vi "Actor Core.vi"(8 "error in":errorcluster, 11 "Nested in":refnum<class "Messages Actor.lvclass">) -> (0 "error out":errorcluster, 3 "Actor out":refnum<class "Actor.lvclass">)   [LabVIEW 2020, in "Messages Actor.lvlib" / "Messages Actor.lvclass"]
doc: "(<B>Filename</B>: Actor Framework.lvlib:Actor.lvclass:Actor Core.vi)\n\nReceives messages to the actor, reacts to them, and initiates any error handling that may shut the actor down.\n\nDescendant classes may override this VI to append parallel tasks for the actor to complete while it handles messages. Overrides use the Call Parent Method node."
uses:
  Messages Actor.lvclass
  C:/Program Files (x86)/National Instruments/LabVIEW 2020/vi.lib/ActorFramework/Actor/Actor.lvclass
  <vilib>/ActorFramework/Actor/Actor.lvclass
  Controls/Language Enum.ctl
  Messages Actor.lvclass/Messages Actor.ctl
  <vilib>/ActorFramework/Actor/Actor.lvclass/Actor.ctl
  <vilib>/ActorFramework/Message Enqueuer/Message Enqueuer.lvclass/Message Enqueuer.ctl
  Write VI Refnum.vi
  <vilib>/ActorFramework/Message Enqueuer/Init from Existing Queue.vi
  <vilib>/ActorFramework/Message Enqueuer/Enqueue.vi
  <vilib>/ActorFramework/Stop Msg/Stop Msg.lvclass
  C:/Program Files (x86)/National Instruments/LabVIEW 2020/vi.lib/ActorFramework/Message/Message.lvclass
  <vilib>/ActorFramework/Message Priority Queue/Priority Enqueue.vi
  <vilib>/ActorFramework/Message Enqueuer/Message Enqueuer.lvclass
panel:
  out "Language":T1
  out "Change":dbl
  out "Status":string
  out "Selected Product":string
  out "Credit":dbl
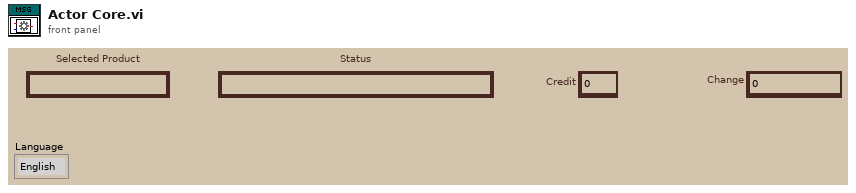
[diagram p1: front panel]
types:
  T1 = typedef "Language Enum.ctl" = enum16{"English", "Español", "Français"}
  T2 = cluster{"Stop":refnum<user-event>, "Language":refnum<user-event>, "Credit":refnum<user-event>, "Status":refnum<user-event>, "Selected Product":refnum<user-event>, "Change":refnum<user-event>}
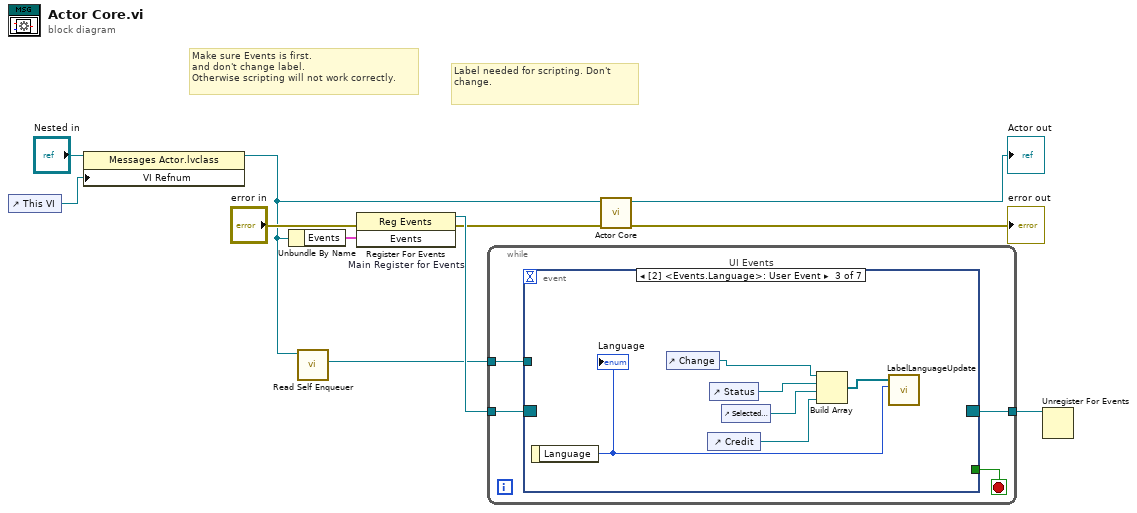
[diagram p0: block diagram]
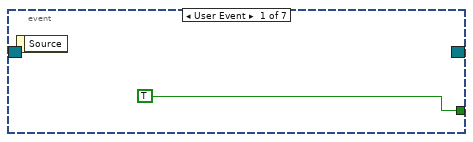
[diagram p2: hidden frame]
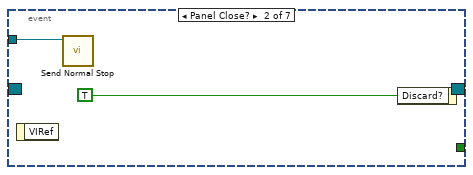
[diagram p3: hidden frame]
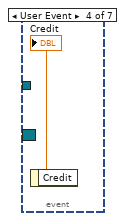
[diagram p4: hidden frame]
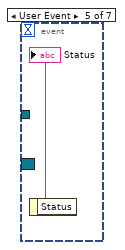
[diagram p5: hidden frame]
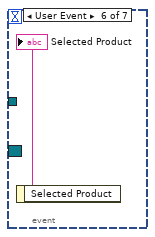
[diagram p6: hidden frame]
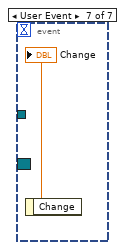
[diagram p7: hidden frame]
diagram:
  # "Label needed for scripting. Don't change."
  # "Make sure Events is first.\nand don't change label.\nOtherwise scripting will not work correctly."
  n1 = control-ref of="This VI"() -> (w1:refnum<vi>)
  n2 = property class="Messages Actor.lvclass"(reference="Nested in", "VI Refnum"=w1) -> (reference out=w2:refnum<class "Messages Actor.lvclass">)  [unwired: 1 in, 1 out]
  n3 = Unbundle By Name(w2) -> ("Events"=w8:T2)
  n4 = call <vilib>:"Read Self Enqueuer.vi"("Actor"=w2) -> ("Self Enqueuer"=w5:refnum<class "Message Enqueuer.lvclass">)  [unwired: 10 in]
  n5 = register-events "Main Register for Events"(error in="error in", w8) -> (reference out=w9:refnum<event-registration>, error out=w3:errorcluster)  [unwired: 1 in]
  n6 = while {
    tunnel: w9 -> [w15]
    tunnel: [w13] -> w7
    tunnel: w5 -> [w12]
    stop <- w14 stop-if-true
    n7 = event "UI Events" shown="[2] <Events.Language>: User Event" {
      selector: w15 -> [_ _ _ _ _ _ _]
      dyn-events: [_ _ _ _ _ _ _] -> w13
      timeout: _ -> [_ _ _ _ _ _ _]
      tunnel: [TRUE _ _ _ _ _ _] -> w14
      tunnel: w12 -> [_ w17 _ _ _ _ _]
      event User Event {
        n8 = event-data() -> ()  [unwired: 1 in, 1 out]
      }
      event Panel Close? {
        n9 = event-data() -> ()  [unwired: 1 in, 1 out]
        n10 = call <vilib>:"Send Normal Stop.vi"("Message Enqueuer"=w17) -> ()  [unwired: 10 in, 1 out]
        n11 = event-data("Discard?"=TRUE) -> ()  [unwired: 1 in, 1 out]
      }
      event User Event {
        n12 = event-data() -> ("Language"=w20:T1)  [unwired: 1 in]
        "Language" <- w20
        n13 = control-ref of="Change"() -> (w19:refnum<vi>)
        n14 = control-ref of="Credit"() -> (w22:refnum<vi>)
        n15 = control-ref of="Status"() -> (w24:refnum<vi>)
        n16 = control-ref of="Selected Product"() -> (w23:refnum<vi>)
        n17 = Build Array(w19, w24, w23, w22) -> (w21:refnum<vi>[])
        n18 = call "LabelLanguageUpdate.vi"("Language"=w20, "Array"=w21) -> ()  [unwired: 10 in]
      }
      event User Event {
        n19 = event-data() -> ("Credit"=→"Credit":dbl)  [unwired: 1 in]
      }
      event User Event {
        n20 = event-data() -> ("Status"=→"Status":string)  [unwired: 1 in]
      }
      event User Event {
        n21 = event-data() -> ("Selected Product"=→"Selected Product":string)  [unwired: 1 in]
      }
      event User Event {
        n22 = event-data() -> ("Change"=→"Change":dbl)  [unwired: 1 in]
      }
    }
  }
  n23 = call-parent "Actor Core.vi"("error in"=w3, "Actor in"=w2) -> ("error out"=→"error out":errorcluster, "Actor out"=→"Actor out":refnum<class "Actor.lvclass">)  [unwired: 8 in]
  n24 = Unregister For Events(event registration refnum=w7) -> ()  [unwired: 1 in, 1 out]
